vi "Octal Channel Write and Read.vi"(0 "hAotfController":u64, 7 "Command":string, 11 "Error In":errorcluster) -> (4 "hAotfController (Dup)":u64, 8 "Response":string, 15 "Error Out":errorcluster)   [LabVIEW 2020]
uses:
  Program Files/Crystal Technology/Developer/AotfLibrary/Dll/AotfLibrary.dll
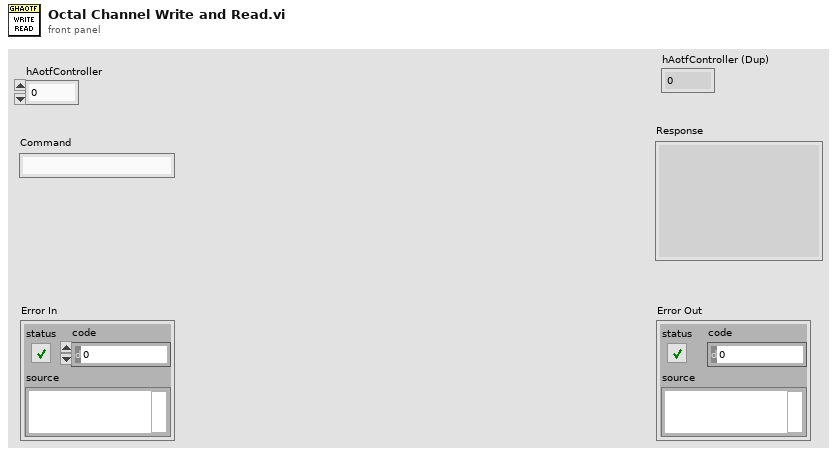
[diagram p1: front panel]
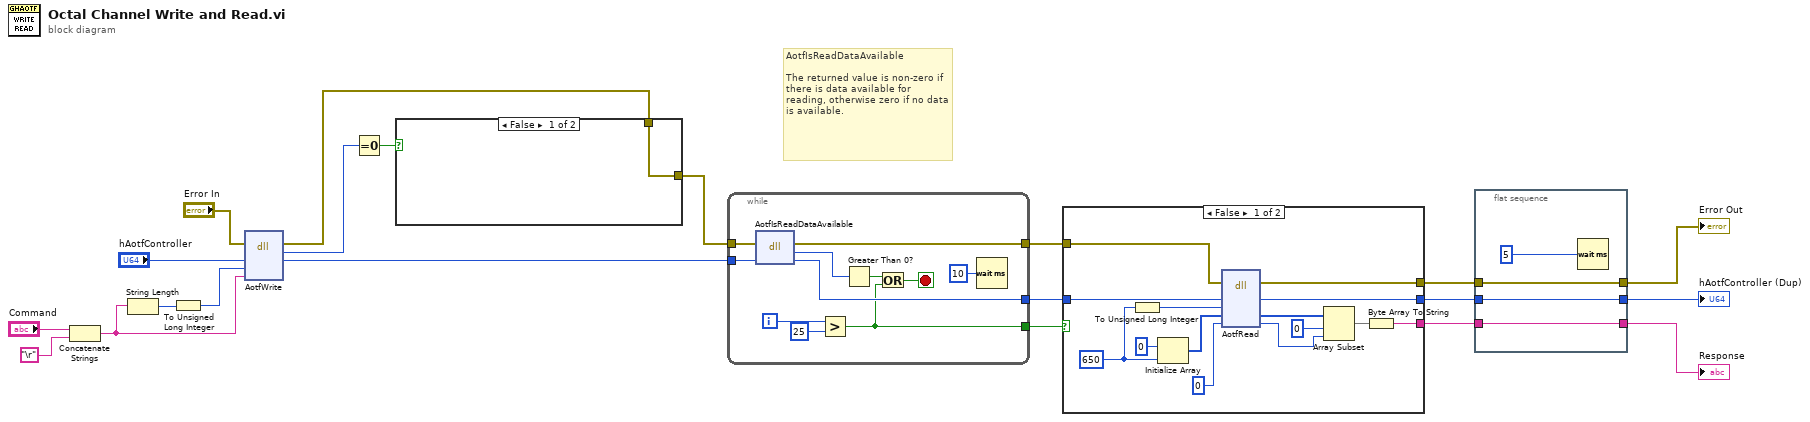
[diagram p0: block diagram]
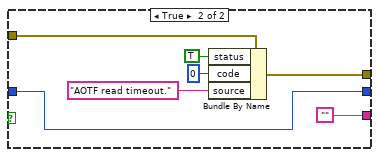
[diagram p2: hidden frame]
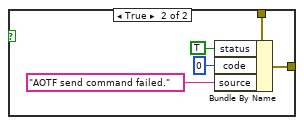
[diagram p3: hidden frame]
diagram:
  # "AotfIsReadDataAvailable\n\nThe returned value is non-zero if there is data available for reading, otherwise zero if no data is available."
  n1 = Concatenate Strings("Command", "\r") -> (w12:string)
  n2 = String Length(string=w12) -> (length=w11:i32)
  n3 = To Unsigned Long Integer(number=w11) -> (unsigned 32bit integer=w10:u32)
  n4 = dll-call lib="C:/Program Files/Crystal Technology/Developer/AotfLibrary/Dll/AotfLibrary.dll" fn="AotfWrite"(error in="Error In", "hAotfController"="hAotfController", "uiLength"=w10, "pData"=w12) -> (error out=w18:errorcluster, "Bool"=w16:u8, "hAotfController"=w19:u64)  [unwired: 4 in, 1 out]
  n5 = Equal To 0?(x=w16) -> (x = 0?=w17:bool)
  n6 = case shown="False" w17 {
    tunnel: w18 -> [w22 w24]
    tunnel: [w22 w23] -> w15
    frame False {
    }
    frame True {
      n7 = Bundle By Name(cluster=w24, "status"=TRUE, "code"=0, "source"="AOTF send command failed.") -> (w23:errorcluster)
    }
  }
  n8 = while {
    tunnel: [w32] -> w7
    tunnel: [w31] -> w9
    tunnel: w19 -> [w30]
    tunnel: [w29] -> w8
    tunnel: w15 -> [w28]
    i -> [w36]
    stop <- w33 stop-if-true
    n9 = dll-call lib="C:/Program Files/Crystal Technology/Developer/AotfLibrary/Dll/AotfLibrary.dll" fn="AotfIsReadDataAvailable"(error in=w28, "hAotfHandle"=w30) -> (error out=w29:errorcluster, "Bool"=w38:u8, "hAotfHandle"=w32:u64)  [unwired: 2 in, 1 out]
    n10 = Greater?(x=w36, y=25) -> (0:w31:bool)
    n11 = Greater Than 0?(x=w38) -> (x > 0?=w34:bool)
    n12 = Or(x=w34, y=w31) -> (x .or. y?=w33:bool)
    n13 = Wait (ms)(milliseconds to wait=u32 10) -> ()  [unwired: 1 out]
  }
  n14 = case shown="False" w9 {
    tunnel: w8 -> [w51 w56]
    tunnel: [w50 w55] -> w6
    tunnel: w7 -> [w52 w54]
    tunnel: [w44 w54] -> w4
    tunnel: [w39 ""] -> w3
    frame False {
      w46 = 650 ("dimension size")
      n15 = To Unsigned Long Integer(number=w46) -> (unsigned 32bit integer=w45:u32)
      n16 = Initialize Array(u8 0 ("element"), w46) -> (w47:u8[])
      n17 = dll-call lib="C:/Program Files/Crystal Technology/Developer/AotfLibrary/Dll/AotfLibrary.dll" fn="AotfRead"(error in=w51, "hAotfHandle"=w52, "uiLength"=w45, "pData"=w47, "puiBytesRead"=0) -> (error out=w50:errorcluster, "hAotfHandle"=w44:u64, "pData"=w43:u8[], "puiBytesRead"=w41:i32)  [unwired: 4 in, 1 out]
      n18 = Array Subset(array=w43, index=0, length=w41) -> (w40:u8[])
      n19 = Byte Array To String(unsigned byte array=w40) -> (string=w39:string)
    }
    frame True {
      n20 = Bundle By Name(cluster=w56, "status"=TRUE, "code"=0, "source"="AOTF read timeout.") -> (w55:errorcluster)
    }
  }
  n21 = flat-sequence {
    tunnel: w6 -> [w63]
    tunnel: [w63] -> w5
    tunnel: w4 -> [w62]
    tunnel: w3 -> [w61]
    tunnel: [w62] -> w2
    tunnel: [w61] -> w1
    frame #0 {
      n22 = Wait (ms)(milliseconds to wait=u32 5) -> ()  [unwired: 1 out]
    }
  }
  "hAotfController (Dup)" <- w2
  "Response" <- w1
  "Error Out" <- w5
